vi "Generate_signal_names_based_on_sensor_names_v2_Core.vi"() -> ()   [LabVIEW 2011]
uses:
  <vilib>/addons/database/Connection.llb/DB Tools Open Connec (String).vi
  <vilib>/addons/database/NI_Database_API.lvlib
panel:
  in  "idtSignal OUT":u16[](array[numeric])=[0, 1, 2, 3, 4, 5, 6, 7, 8, 9, 10, 11, 12, 13, 14, 15, 16, 17, 18, 19, 20, 21, 22, 23, 24, 25, 26, 27, 28, 29, 30, 31, 32, 33, 34, 35, 36, 37, 38, 39, 40, 41, 42, 43, 44, 45, 46, 47, 48, 49, 50, 51, 52, 53, 54, 55, 56, 57, 58, 59, 60, 61, 62, 63, 64, 65, 66, 67, 68, 69, 70, 71, 72, 73, 74, 75, 76, 77, 78, 79, 80, 81, 82, 83, 84, 85, 86, 87, 88, 89, 90, 91, 92, 93, 94, 95, 96, 97, 98, 99, 100, 101, 102, 103, 104, 105, 106, 107, 108, 109, 110, 111, 112, 113, 114, 115, 116, 117, 118, 119, 120, 121, 122, 123, 124, 125, 126, 127, 128, 129, 130, 131, 132, 133, 134, 135, 136, 137, 138, 139, 140, 141, 142, 143, 144, 145, 146, 147, 148, 149, 150, 151, 152, 153, 154, 155, 156, 157, 158, 159, 160, 161, 162, 163, 164, 165, 166, 167, 168, 169, 170, 171, 172, 173, 174, 175, 176, 177, 178, 179, 180, 181, 182, 183, 184, 185, 186, 187, 188, 189, 190, 191, 192, 193, 194, 195, 196, 197, 198, 199, 200, 201, 202, 203, 204, 205, 206, 207, 208, 209, 210, 211, 212, 213, 214, 215, 216, 217, 218, 219, 220, 221, 222, 223, 224, 225, 226, 227, 228, 229, 230, 231, 232, 233, 234, 235, 236, 237, 238, 239, 240, 241, 242, 243, 244, 245, 246, 247, 248, 249, 250, 251, 252, 253, 254, 255, 256, 257, 258, 259, 260, 261, 262, 263, 264, 265, 266, 267, 268, 269, 270, 271, 272, 273, 274, 275, 276, 277, 278, 279, 280, 281, 282, 283, 284, 285, 286, 287, 288, 289, 290, 291, 292, 293, 294, 295, 296, 297, 298, 299, 300, 301, 302, 303, 304, 305, 306, 307, 308, 309, 310, 311, 312, 313, 314, 315, 316, 317, 318, 319, 320, 321, 322, 323, 324, 325, 326, 327, 328, 329, 330, 331, 332, 333, 334, 335, 336, 337, 338, 339, 340, 341, 342, 343, 344, 345, 346, 347, 348, 349, 350, 351, 352, 353, 354, 355, 356, 357, 358, 359, 360, 361, 362, 363, 364, 365, 366, 367, 368, 369, 370, 371, 372, 373, 374, 375, 376, 377, 378, 379, 380, 381, 382, 383, 384, 385, 386, 387, 388, 389, 390, 391, 392, 393, 394, 395, 396, 397, 398, 399, 400, 401, 402, 403, 404, 405, 406, 407, 408, 409, 410, 411, 412, 413, 414, 415, 416, 417, 418, 419, 420, 421, 422, 423, 424, 425, 426, 427, 428, 429, 430, 431, 432, 433, 434, 435, 437]
  out "error out":errorcluster={"status"=TRUE, "code"=-2147217900, "source"="NI_Database_API.lvlib:Cmd Execute.vi->NI_Database_API.lvlib:DB Tools Insert Data.vi->Generate_signal_names_based_on_sensor_names_v2_Erraring.vi<ERR>ADO Error: 0x80040E14\r\nException occured in Microsoft OLE DB Provider for ODBC Drivers: [MySQL][ODBC 5.1 Driver][mysqld-5.5.15]Duplicate entry '428' for key 'PRIMARY' in NI_Database_API.lvlib:Rec Create - Command.vi->NI_Database_API.lvlib:Cmd Execute.vi->NI_Database_API.lvlib:DB Tools Insert Data.vi->Generate_signal_names_based_on_sensor_names_v2_Erraring.vi"}
  in  "SignalNames":string[](array[string])=["Hitrost vrtenja 0 .RotSpeed.[1 impulz po obratu]", "Hitrost vrtenja 0 .DC.[V]", "Hitrost vrtenja 1 .RotSpeed.[100Hz]", "Hitrost vrtenja 1 .DC.[V]", "Relativne vibracije ZKL1 .s1.00A.[um]", "Relativne vibracije ZKL1 .s1.00Ph.[°]", "Relativne vibracije ZKL1 .s2.00A.[um]", "Relativne vibracije ZKL1 .s2.00Ph.[°]", "Relativne vibracije ZKL1 .s3.00A.[um]", "Relativne vibracije ZKL1 .s3.00Ph.[°]", "Relativne vibracije ZKL1 .Rest.[um]", "Relativne vibracije ZKL1 .DC.[um]", "Relativne vibracije ZKL1 .EqPeak.[um]", "Relativne vibracije ZKL1 &Relativne vibracije ZKL2 .Smax.[um]", "Relativne vibracije ZKL2 .s1.00A.[um]", "Relativne vibracije ZKL2 .s1.00Ph.[°]", "Relativne vibracije ZKL2 .s2.00A.[um]", "Relativne vibracije ZKL2 .s2.00Ph.[°]", "Relativne vibracije ZKL2 .s3.00A.[um]", "Relativne vibracije ZKL2 .s3.00Ph.[°]", "Relativne vibracije ZKL2 .Rest.[um]", "Relativne vibracije ZKL2 .DC.[um]", "Relativne vibracije ZKL2 .EqPeak.[um]", "Relativne vibracije SVL1 .s1.00A.[um]", "Relativne vibracije SVL1 .s1.00Ph.[°]", "Relativne vibracije SVL1 .s2.00A.[um]", "Relativne vibracije SVL1 .s2.00Ph.[°]", "Relativne vibracije SVL1 .s3.00A.[um]", "Relativne vibracije SVL1 .s3.00Ph.[°]", "Relativne vibracije SVL1 .Rest.[um]", "Relativne vibracije SVL1 .DC.[um]", "Relativne vibracije SVL1 .EqPeak.[um]", "Relativne vibracije SVL1 &Relativne vibracije SVL2 .Smax.[um]", "Relativne vibracije SVL2 .s1.00A.[um]", "Relativne vibracije SVL2 .s1.00Ph.[°]", "Relativne vibracije SVL2 .s2.00A.[um]", "Relativne vibracije SVL2 .s2.00Ph.[°]", "Relativne vibracije SVL2 .s3.00A.[um]", "Relativne vibracije SVL2 .s3.00Ph.[°]", "Relativne vibracije SVL2 .Rest.[um]", "Relativne vibracije SVL2 .DC.[um]", "Relativne vibracije SVL2 .EqPeak.[um]", "Relativne vibracije VVL1 .s1.00A.[um]", "Relativne vibracije VVL1 .s1.00Ph.[°]", "Relativne vibracije VVL1 .s2.00A.[um]", "Relativne vibracije VVL1 .s2.00Ph.[°]", "Relativne vibracije VVL1 .s3.00A.[um]", "Relativne vibracije VVL1 .s3.00Ph.[°]", "Relativne vibracije VVL1 .Rest.[um]", "Relativne vibracije VVL1 .DC.[um]", "Relativne vibracije VVL1 .EqPeak.[um]", "Relativne vibracije VVL1 &Relativne vibracije VVL2 .Smax.[um]", "Relativne vibracije VVL2 .s1.00A.[um]", "Relativne vibracije VVL2 .s1.00Ph.[°]", "Relativne vibracije VVL2 .s2.00A.[um]", "Relativne vibracije VVL2 .s2.00Ph.[°]", "Relativne vibracije VVL2 .s3.00A.[um]", "Relativne vibracije VVL2 .s3.00Ph.[°]", "Relativne vibracije VVL2 .Rest.[um]", "Relativne vibracije VVL2 .DC.[um]", "Relativne vibracije VVL2 .EqPeak.[um]", "Relativne vibracije TVL1 .s1.00A.[um]", "Relativne vibracije TVL1 .s1.00Ph.[°]", "Relativne vibracije TVL1 .s2.00A.[um]", "Relativne vibracije TVL1 .s2.00Ph.[°]", "Relativne vibracije TVL1 .s3.00A.[um]", "Relativne vibracije TVL1 .s3.00Ph.[°]", "Relativne vibracije TVL1 .Rest.[um]", "Relativne vibracije TVL1 .DC.[um]", "Relativne vibracije TVL1 .EqPeak.[um]", "Relativne vibracije TVL1 &Relativne vibracije TVL2 .Smax.[um]", "Relativne vibracije TVL2 .s1.00A.[um]", "Relativne vibracije TVL2 .s1.00Ph.[°]", "Relativne vibracije TVL2 .s2.00A.[um]", "Relativne vibracije TVL2 .s2.00Ph.[°]", "Relativne vibracije TVL2 .s3.00A.[um]", "Relativne vibracije TVL2 .s3.00Ph.[°]", "Relativne vibracije TVL2 .Rest.[um]", "Relativne vibracije TVL2 .DC.[um]", "Relativne vibracije TVL2 .EqPeak.[um]", "Absolutne vibracije ZKL1 .s1.00A.[mm/s]", "Absolutne vibracije ZKL1 .s1.00Ph.[°]", "Absolutne vibracije ZKL1 .s2.00A.[mm/s]", "Absolutne vibracije ZKL1 .s2.00Ph.[°]", "Absolutne vibracije ZKL1 .s3.00A.[mm/s]", "Absolutne vibracije ZKL1 .s3.00Ph.[°]", "Absolutne vibracije ZKL1 .Rest.[mm/s]", "Absolutne vibracije ZKL1 .RMS.[mm/s]", "Absolutne vibracije ZKL1 .DC.[mm/s]", "Absolutne vibracije ZKL2 .s1.00A.[mm/s]", "Absolutne vibracije ZKL2 .s1.00Ph.[°]", "Absolutne vibracije ZKL2 .s2.00A.[mm/s]", "Absolutne vibracije ZKL2 .s2.00Ph.[°]", "Absolutne vibracije ZKL2 .s3.00A.[mm/s]", "Absolutne vibracije ZKL2 .s3.00Ph.[°]", "Absolutne vibracije ZKL2 .Rest.[mm/s]", "Absolutne vibracije ZKL2 .RMS.[mm/s]", "Absolutne vibracije ZKL2 .DC.[mm/s]", "Absolutne vibracije SVL1 .s1.00A.[mm/s]", "Absolutne vibracije SVL1 .s1.00Ph.[°]", "Absolutne vibracije SVL1 .s2.00A.[mm/s]", "Absolutne vibracije SVL1 .s2.00Ph.[°]", "Absolutne vibracije SVL1 .s3.00A.[mm/s]", "Absolutne vibracije SVL1 .s3.00Ph.[°]", "Absolutne vibracije SVL1 .Rest.[mm/s]", "Absolutne vibracije SVL1 .RMS.[mm/s]", "Absolutne vibracije SVL1 .DC.[mm/s]", "Absolutne vibracije SVL2 .s1.00A.[mm/s]", "Absolutne vibracije SVL2 .s1.00Ph.[°]", "Absolutne vibracije SVL2 .s2.00A.[mm/s]", "Absolutne vibracije SVL2 .s2.00Ph.[°]", "Absolutne vibracije SVL2 .s3.00A.[mm/s]", "Absolutne vibracije SVL2 .s3.00Ph.[°]", "Absolutne vibracije SVL2 .Rest.[mm/s]", "Absolutne vibracije SVL2 .RMS.[mm/s]", "Absolutne vibracije SVL2 .DC.[mm/s]", "Absolutne vibracije VVL1 .s1.00A.[mm/s]", "Absolutne vibracije VVL1 .s1.00Ph.[°]", "Absolutne vibracije VVL1 .s2.00A.[mm/s]", "Absolutne vibracije VVL1 .s2.00Ph.[°]", "Absolutne vibracije VVL1 .s3.00A.[mm/s]", "Absolutne vibracije VVL1 .s3.00Ph.[°]", "Absolutne vibracije VVL1 .Rest.[mm/s]", "Absolutne vibracije VVL1 .RMS.[mm/s]", "Absolutne vibracije VVL1 .DC.[mm/s]", "Absolutne vibracije VVL1 .s1.00A.[mm/s]", "Absolutne vibracije VVL1 .s1.00Ph.[°]", "Absolutne vibracije VVL1 .s2.00A.[mm/s]", "Absolutne vibracije VVL1 .s2.00Ph.[°]", "Absolutne vibracije VVL1 .s3.00A.[mm/s]", "Absolutne vibracije VVL1 .s3.00Ph.[°]", "Absolutne vibracije VVL1 .Rest.[mm/s]", "Absolutne vibracije VVL1 .RMS.[mm/s]", "Absolutne vibracije VVL1 .DC.[mm/s]", "Absolutne vibracije TVL1 .s1.00A.[mm/s]", "Absolutne vibracije TVL1 .s1.00Ph.[°]", "Absolutne vibracije TVL1 .s2.00A.[mm/s]", "Absolutne vibracije TVL1 .s2.00Ph.[°]", "Absolutne vibracije TVL1 .s3.00A.[mm/s]", "Absolutne vibracije TVL1 .s3.00Ph.[°]", "Absolutne vibracije TVL1 .Rest.[mm/s]", "Absolutne vibracije TVL1 .RMS.[mm/s]", "Absolutne vibracije TVL1 .DC.[mm/s]", "Absolutne vibracije TVL2 .s1.00A.[mm/s]", "Absolutne vibracije TVL2 .s1.00Ph.[°]", "Absolutne vibracije TVL2 .s2.00A.[mm/s]", "Absolutne vibracije TVL2 .s2.00Ph.[°]", "Absolutne vibracije TVL2 .s3.00A.[mm/s]", "Absolutne vibracije TVL2 .s3.00Ph.[°]", "Absolutne vibracije TVL2 .Rest.[mm/s]", "Absolutne vibracije TVL2 .RMS.[mm/s]", "Absolutne vibracije TVL2 .DC.[mm/s]", "Aksialni pomik  AxP1 .DC.[um]", "Aksialni pomik  AxP2 .DC.[um]", "Absolutne vibracije paketa VP1 .RMS.[mm/s]", "Absolutne vibracije paketa VP1 .s20.00A.[mm/s]", "Absolutne vibracije paketa VP1 .s40.00A.[mm/s]", "Absolutne vibracije paketa VP1 .s60.00A.[mm/s]", "Absolutne vibracije paketa VP1 .Rest.[mm/s]", "Absolutne vibracije paketa VP2 .RMS.[mm/s]", "Absolutne vibracije paketa VP2 .s20.00A.[mm/s]", "Absolutne vibracije paketa VP2 .s40.00A.[mm/s]", "Absolutne vibracije paketa VP2 .s60.00A.[mm/s]", "Absolutne vibracije paketa VP2 .Rest.[mm/s]", "Zracna reža zgoraj, dajalec 1 .MinPole01.[mm]", "Zracna reža zgoraj, dajalec 1 .MinPole02.[mm]", "Zracna reža zgoraj, dajalec 1 .MinPole03.[mm]", "Zracna reža zgoraj, dajalec 1 .MinPole04.[mm]", "Zracna reža zgoraj, dajalec 1 .MinPole05.[mm]", "Zracna reža zgoraj, dajalec 1 .MinPole06.[mm]", "Zracna reža zgoraj, dajalec 1 .MinPole07.[mm]", "Zracna reža zgoraj, dajalec 1 .MinPole08.[mm]", "Zracna reža zgoraj, dajalec 1 .MinPole09.[mm]", "Zracna reža zgoraj, dajalec 1 .MinPole10.[mm]", "Zracna reža zgoraj, dajalec 1 .MinPole11.[mm]", "Zracna reža zgoraj, dajalec 1 .MinPole12.[mm]", "Zracna reža zgoraj, dajalec 1 .MinPole13.[mm]", "Zracna reža zgoraj, dajalec 1 .MinPole14.[mm]", "Zracna reža zgoraj, dajalec 1 .MinPole15.[mm]", "Zracna reža zgoraj, dajalec 1 .MinPole16.[mm]", "Zracna reža zgoraj, dajalec 1 .MinPole17.[mm]", "Zracna reža zgoraj, dajalec 1 .MinPole18.[mm]", "Zracna reža zgoraj, dajalec 1 .MinPole19.[mm]", "Zracna reža zgoraj, dajalec 1 .MinPole20.[mm]", "Zracna reža zgoraj, dajalec 1 .MinExtremaMin.[mm]", "Zracna reža zgoraj, dajalec 1 .MinExtremaMinPoleNum.[Number]", "Zracna reža zgoraj, dajalec 1 .MaxExtremaMin.[mm]", "Zracna reža zgoraj, dajalec 1 .MaxExtremaMinPoleNum.[Number]", "Zracna reža zgoraj, dajalec 1 .DCExtremaMin.[mm]", "Zracna reža zgoraj, dajalec 1 .MaxDiff.[mm]", "Zracna reža zgoraj, dajalec 1 .MaxDiffPoleNum.[Number]", "Zracna reža zgoraj, dajalec 1 .Max Diff Pole Number.[mm]", "Zracna reža zgoraj, dajalec 1 .s1.00A.[mm]", "Zracna reža zgoraj, dajalec 1 .s1.00Ph.[°]", "Zracna reža zgoraj, dajalec 1 .s2.00A.[mm]", "Zracna reža zgoraj, dajalec 1 .s2.00Ph.[°]", "Zracna reža zgoraj, dajalec 1 .DC.[mm]", "Zracna reža zgoraj, dajalec 2 .MinPole01.[mm]", "Zracna reža zgoraj, dajalec 2 .MinPole02.[mm]", "Zracna reža zgoraj, dajalec 2 .MinPole03.[mm]", "Zracna reža zgoraj, dajalec 2 .MinPole04.[mm]", "Zracna reža zgoraj, dajalec 2 .MinPole05.[mm]", "Zracna reža zgoraj, dajalec 2 .MinPole06.[mm]", "Zracna reža zgoraj, dajalec 2 .MinPole07.[mm]", "Zracna reža zgoraj, dajalec 2 .MinPole08.[mm]", "Zracna reža zgoraj, dajalec 2 .MinPole09.[mm]", "Zracna reža zgoraj, dajalec 2 .MinPole10.[mm]", "Zracna reža zgoraj, dajalec 2 .MinPole11.[mm]", "Zracna reža zgoraj, dajalec 2 .MinPole12.[mm]", "Zracna reža zgoraj, dajalec 2 .MinPole13.[mm]", "Zracna reža zgoraj, dajalec 2 .MinPole14.[mm]", "Zracna reža zgoraj, dajalec 2 .MinPole15.[mm]", "Zracna reža zgoraj, dajalec 2 .MinPole16.[mm]", "Zracna reža zgoraj, dajalec 2 .MinPole17.[mm]", "Zracna reža zgoraj, dajalec 2 .MinPole18.[mm]", "Zracna reža zgoraj, dajalec 2 .MinPole19.[mm]", "Zracna reža zgoraj, dajalec 2 .MinPole20.[mm]", "Zracna reža zgoraj, dajalec 2 .MinExtremaMin.[mm]", "Zracna reža zgoraj, dajalec 2 .MinExtremaMinPoleNum.[Number]", "Zracna reža zgoraj, dajalec 2 .MaxExtremaMin.[mm]", "Zracna reža zgoraj, dajalec 2 .MaxExtremaMinPoleNum.[Number]", "Zracna reža zgoraj, dajalec 2 .DCExtremaMin.[mm]", "Zracna reža zgoraj, dajalec 2 .MaxDiff.[mm]", "Zracna reža zgoraj, dajalec 2 .MaxDiffPoleNum.[Number]", "Zracna reža zgoraj, dajalec 2 .Max Diff Pole Number.[mm]", "Zracna reža zgoraj, dajalec 2 .s1.00A.[mm]", "Zracna reža zgoraj, dajalec 2 .s1.00Ph.[°]", "Zracna reža zgoraj, dajalec 2 .s2.00A.[mm]", "Zracna reža zgoraj, dajalec 2 .s2.00Ph.[°]", "Zracna reža zgoraj, dajalec 2 .DC.[mm]", "Magnetno polje, dajalec zgoraj .MaxPole01.[T]", "Magnetno polje, dajalec zgoraj .MaxPole02.[T]", "Magnetno polje, dajalec zgoraj .MaxPole03.[T]", "Magnetno polje, dajalec zgoraj .MaxPole04.[T]", "Magnetno polje, dajalec zgoraj .MaxPole05.[T]", "Magnetno polje, dajalec zgoraj .MaxPole06.[T]", "Magnetno polje, dajalec zgoraj .MaxPole07.[T]", "Magnetno polje, dajalec zgoraj .MaxPole08.[T]", "Magnetno polje, dajalec zgoraj .MaxPole09.[T]", "Magnetno polje, dajalec zgoraj .MaxPole10.[T]", "Magnetno polje, dajalec zgoraj .MaxPole11.[T]", "Magnetno polje, dajalec zgoraj .MaxPole12.[T]", "Magnetno polje, dajalec zgoraj .MaxPole13.[T]", "Magnetno polje, dajalec zgoraj .MaxPole14.[T]", "Magnetno polje, dajalec zgoraj .MaxPole15.[T]", "Magnetno polje, dajalec zgoraj .MaxPole16.[T]", "Magnetno polje, dajalec zgoraj .MaxPole17.[T]", "Magnetno polje, dajalec zgoraj .MaxPole18.[T]", "Magnetno polje, dajalec zgoraj .MaxPole19.[T]", "Magnetno polje, dajalec zgoraj .MaxPole20.[T]", "Magnetno polje, dajalec zgoraj .MinExtremaMax.[T]", "Magnetno polje, dajalec zgoraj .MinExtremaMaxPoleNum.[Number]", "Magnetno polje, dajalec zgoraj .MaxExtremaMax.[T]", "Magnetno polje, dajalec zgoraj .MaxExtremaMaxPoleNum.[Number]", "Magnetno polje, dajalec zgoraj .DCExtremaMax.[T]", "Magnetno polje, dajalec zgoraj .MaxDiff.[T]", "Magnetno polje, dajalec zgoraj .MaxDiffPoleNum.[Number]", "Magnetno polje, dajalec zgoraj .Max Diff Pole Number.[T]", "Hitrost vrtenja 1 &Napetost generatorja faza R .LoadAngleDelta.[100Hz]", "Napetost generatorja faza R - G1 .ActivePowerIntegration.[kV]", "Napetost generatorja faza R - G1 .ReactivePowerIntegration.[kV]", "Napetost generatorja faza R - G1 .ApparentPower.[kV]", "Napetost generatorja faza R - G1 .Ampl@Freq.[kV]", "Napetost generatorja faza S - G1 .Ampl@Freq.[kV]", "Napetost generatorja faza T - G1 .Ampl@Freq.[kV]", "Tok generatorja faza R - G1 .Ampl@Freq.[kA]", "Tok generatorja faza S - G1 .Ampl@Freq.[kA]", "Tok generatorja faza T - G1 .Ampl@Freq.[kA]", "Napetost za blok transformatorjem faza R - G1 .Ampl@Freq.[kV]", "Napetost za blok transformatorjem faza S - G1 .Ampl@Freq.[kV]", "Napetost za blok transformatorjem faza T - G1 .Ampl@Freq.[kV]", "Tok za blok transformatorjem faza R - G1 .Ampl@Freq.[A]", "Tok za blok transformatorjem faza S - G1 .Ampl@Freq.[A]", "Tok za blok transformatorjem faza T - G1 .Ampl@Freq.[A]", "Napetost generatorja faza R - G1 .SignalFrequency.[Hz]", "Napetost generatorja faza S - G1 .SignalFrequency.[Hz]", "Napetost generatorja faza T - G1 .SignalFrequency.[Hz]", "Tok generatorja faza R - G1 .SignalFrequency.[Hz]", "Tok generatorja faza S - G1 .SignalFrequency.[Hz]", "Tok generatorja faza T - G1 .SignalFrequency.[Hz]", "Napetost za blok transformatorjem faza R - G1 .SignalFrequency.[Hz]", "Napetost za blok transformatorjem faza S - G1 .SignalFrequency.[Hz]", "Napetost za blok transformatorjem faza T - G1 .SignalFrequency.[Hz]", "Tok za blok transformatorjem faza R - G1 .SignalFrequency.[Hz]", "Tok za blok transformatorjem faza S - G1 .SignalFrequency.[Hz]", "Tok za blok transformatorjem faza T - G1 .SignalFrequency.[Hz]", "Napetost generatorja faza R - G1 .THD.[%]", "Napetost generatorja faza S - G1 .THD.[%]", "Napetost generatorja faza T - G1 .THD.[%]", "Tok generatorja faza R - G1 .THD.[%]", "Tok generatorja faza S - G1 .THD.[%]", "Tok generatorja faza T - G1 .THD.[%]", "Napetost za blok transformatorjem faza R - G1 .THD.[%]", "Napetost za blok transformatorjem faza S - G1 .THD.[%]", "Napetost za blok transformatorjem faza T - G1 .THD.[%]", "Tok za blok transformatorjem faza R - G1 .THD.[%]", "Tok za blok transformatorjem faza S - G1 .THD.[%]", "Tok za blok transformatorjem faza T - G1 .THD.[%]", "Napetost generatorja faza R - G1 &Napetost generatorja faza S - G1 .PhaseDifference.[°]", "Napetost generatorja faza S - G1 &Napetost generatorja faza T - G1 .PhaseDifference.[°]", "Napetost generatorja faza T - G1 &Napetost generatorja faza R - G1 .PhaseDifference.[°]", "Tok generatorja faza R - G1 &Tok generatorja faza S - G1 .PhaseDifference.[°]", "Tok generatorja faza S - G1 &Tok generatorja faza T - G1 .PhaseDifference.[°]", "Tok generatorja faza T - G1 &Tok generatorja faza R - G1 .PhaseDifference.[°]", "Napetost za blok transformatorjem faza R - G1 &Napetost za blok transformatorjem faza S - G1 .PhaseDifference.[°]", "Napetost za blok transformatorjem faza S - G1 &Napetost za blok transformatorjem faza T - G1 .PhaseDifference.[°]", "Napetost za blok transformatorjem faza T - G1 &Napetost za blok transformatorjem faza R - G1 .PhaseDifference.[°]", "Tok za blok transformatorjem faza R - G1 &Tok za blok transformatorjem faza S - G1 .PhaseDifference.[°]", "Tok za blok transformatorjem faza S - G1 &Tok za blok transformatorjem faza T - G1 .PhaseDifference.[°]", "Tok za blok transformatorjem faza T - G1 &Tok za blok transformatorjem faza R - G1 .PhaseDifference.[°]", "Napetost generatorja faza R - G1 .CosFi.[%]", "Napetost generatorja faza R - G1 .TotalTHD.[%]", "Tok generatorja faza R - G1 .TotalTHD.[%]", "Napetost za blok transformatorjem faza R - G1 .TotalTHD.[%]", "Tok za blok transformatorjem faza R - G1 .TotalTHD.[%]", "ModbusData_000", "ModbusData_001", "ModbusData_002", "ModbusData_003", "ModbusData_004", "ModbusData_005", "ModbusData_006", "ModbusData_007", "ModbusData_008", "ModbusData_009", "ModbusData_010", "ModbusData_011", "ModbusData_012", "ModbusData_013", "ModbusData_014", "ModbusData_015", "ModbusData_016", "ModbusData_017", "ModbusData_018", "ModbusData_019", "ModbusData_020", "ModbusData_021", "ModbusData_022", "ModbusData_023", "ModbusData_024", "ModbusData_025", "ModbusData_026", "ModbusData_027", "ModbusData_028", "ModbusData_029", "ModbusData_030", "ModbusData_031", "ModbusData_032", "ModbusData_033", "ModbusData_034", "ModbusData_035", "ModbusData_036", "ModbusData_037", "ModbusData_038", "ModbusData_039", "ModbusData_040", "ModbusData_041", "ModbusData_042", "ModbusData_043", "ModbusData_044", "ModbusData_045", "ModbusData_046", "ModbusData_047", "ModbusData_048", "ModbusData_049", "ModbusData_050", "ModbusData_051", "ModbusData_052", "ModbusData_053", "ModbusData_054", "ModbusData_055", "ModbusData_056", "ModbusData_057", "ModbusData_058", "ModbusData_059", "ModbusData_060", "ModbusData_061", "ModbusData_062", "ModbusData_063", "ModbusData_064", "ModbusData_065", "ModbusData_066", "ModbusData_067", "ModbusData_068", "ModbusData_069", "ModbusData_070", "ModbusData_071", "ModbusData_072", "ModbusData_073", "ModbusData_074", "ModbusData_075", "ModbusData_076", "ModbusData_077", "ModbusData_078", "ModbusData_079", "ModbusData_080", "ModbusData_081", "ModbusData_082", "ModbusData_083", "ModbusData_084", "ModbusData_085", "ModbusData_086", "ModbusData_087", "ModbusData_088", "ModbusData_089", "ModbusData_090", "ModbusData_091", "ModbusData_092", "ModbusData_093", "ModbusData_094", "ModbusData_095", "ModbusData_096", "ModbusData_097", "ModbusData_098", "ModbusData_099", "Absolutne vibracije paketa VP1 .DC.[mm/s]", "Absolutne vibracije paketa VP2 .DC.[mm/s]", "Absolutne vibracije paketa VP1 .EqPeak.[mm/s]", "Absolutne vibracije paketa VP2 .EqPeak.[mm/s]", "Magnetno polje, dajalec zgoraj .DC.[T]", "Absolutne vibracije ZKL1 .EqPeak.[mm/s]", "Absolutne vibracije ZKL2 .EqPeak.[mm/s]", "Absolutne vibracije SVL1 .EqPeak.[mm/s]", "Absolutne vibracije SVL2 .EqPeak.[mm/s]", "Absolutne vibracije VVL1 .EqPeak.[mm/s]", "Absolutne vibracije VVL1 .EqPeak.[mm/s]", "Absolutne vibracije TVL1 .EqPeak.[mm/s]", "Absolutne vibracije TVL2 .EqPeak.[mm/s]", "Magnetno polje, dajalec zgoraj .EqPeak.[T]", "Relativne vibracije ZKL1 &Relativne vibracije ZKL2 .SP2Pmax.[um]", "Relativne vibracije SVL1 &Relativne vibracije SVL2 .SP2Pmax.[um]", "Relativne vibracije VVL1 &Relativne vibracije VVL2 .SP2Pmax.[um]", "Relativne vibracije TVL1 &Relativne vibracije TVL2 .SP2Pmax.[um]", "Magnetno polje, dajalec zgoraj .RMS.[T]", "Magnetno polje, dajalec zgoraj .EqPeak.[T]", "Napetost generatorja faza R .s10.00A.[kV]", "Napetost generatorja faza R .s10.00Ph.[°]"]
  in  "SignalLabels":string[](array[string])=["TRG000.RotSpeed", "TRG000.DC", "TRG001.RotSpeed", "TRG001.DC", "RV000.s1.00A", "RV000.s1.00Ph", "RV000.s2.00A", "RV000.s2.00Ph", "RV000.s3.00A", "RV000.s3.00Ph", "RV000.Rest", "RV000.DC", "RV000.EqPeak", "RV000&RV001.Smax", "RV001.s1.00A", "RV001.s1.00Ph", "RV001.s2.00A", "RV001.s2.00Ph", "RV001.s3.00A", "RV001.s3.00Ph", "RV001.Rest", "RV001.DC", "RV001.EqPeak", "RV002.s1.00A", "RV002.s1.00Ph", "RV002.s2.00A", "RV002.s2.00Ph", "RV002.s3.00A", "RV002.s3.00Ph", "RV002.Rest", "RV002.DC", "RV002.EqPeak", "RV002&RV003.Smax", "RV003.s1.00A", "RV003.s1.00Ph", "RV003.s2.00A", "RV003.s2.00Ph", "RV003.s3.00A", "RV003.s3.00Ph", "RV003.Rest", "RV003.DC", "RV003.EqPeak", "RV004.s1.00A", "RV004.s1.00Ph", "RV004.s2.00A", "RV004.s2.00Ph", "RV004.s3.00A", "RV004.s3.00Ph", "RV004.Rest", "RV004.DC", "RV004.EqPeak", "RV004&RV005.Smax", "RV005.s1.00A", "RV005.s1.00Ph", "RV005.s2.00A", "RV005.s2.00Ph", "RV005.s3.00A", "RV005.s3.00Ph", "RV005.Rest", "RV005.DC", "RV005.EqPeak", "RV006.s1.00A", "RV006.s1.00Ph", "RV006.s2.00A", "RV006.s2.00Ph", "RV006.s3.00A", "RV006.s3.00Ph", "RV006.Rest", "RV006.DC", "RV006.EqPeak", "RV006&RV007.Smax", "RV007.s1.00A", "RV007.s1.00Ph", "RV007.s2.00A", "RV007.s2.00Ph", "RV007.s3.00A", "RV007.s3.00Ph", "RV007.Rest", "RV007.DC", "RV007.EqPeak", "AV000.s1.00A", "AV000.s1.00Ph", "AV000.s2.00A", "AV000.s2.00Ph", "AV000.s3.00A", "AV000.s3.00Ph", "AV000.Rest", "AV000.RMS", "AV000.DC", "AV001.s1.00A", "AV001.s1.00Ph", "AV001.s2.00A", "AV001.s2.00Ph", "AV001.s3.00A", "AV001.s3.00Ph", "AV001.Rest", "AV001.RMS", "AV001.DC", "AV002.s1.00A", "AV002.s1.00Ph", "AV002.s2.00A", "AV002.s2.00Ph", "AV002.s3.00A", "AV002.s3.00Ph", "AV002.Rest", "AV002.RMS", "AV002.DC", "AV003.s1.00A", "AV003.s1.00Ph", "AV003.s2.00A", "AV003.s2.00Ph", "AV003.s3.00A", "AV003.s3.00Ph", "AV003.Rest", "AV003.RMS", "AV003.DC", "AV004.s1.00A", "AV004.s1.00Ph", "AV004.s2.00A", "AV004.s2.00Ph", "AV004.s3.00A", "AV004.s3.00Ph", "AV004.Rest", "AV004.RMS", "AV004.DC", "AV005.s1.00A", "AV005.s1.00Ph", "AV005.s2.00A", "AV005.s2.00Ph", "AV005.s3.00A", "AV005.s3.00Ph", "AV005.Rest", "AV005.RMS", "AV005.DC", "AV006.s1.00A", "AV006.s1.00Ph", "AV006.s2.00A", "AV006.s2.00Ph", "AV006.s3.00A", "AV006.s3.00Ph", "AV006.Rest", "AV006.RMS", "AV006.DC", "AV007.s1.00A", "AV007.s1.00Ph", "AV007.s2.00A", "AV007.s2.00Ph", "AV007.s3.00A", "AV007.s3.00Ph", "AV007.Rest", "AV007.RMS", "AV007.DC", "AXD000.DC", "AXD001.DC", "AV008.RMS", "AV008.s20.00A", "AV008.s40.00A", "AV008.s60.00A", "AV008.Rest", "AV009.RMS", "AV009.s20.00A", "AV009.s40.00A", "AV009.s60.00A", "AV009.Rest", "AG000.MinPole01", "AG000.MinPole02", "AG000.MinPole03", "AG000.MinPole04", "AG000.MinPole05", "AG000.MinPole06", "AG000.MinPole07", "AG000.MinPole08", "AG000.MinPole09", "AG000.MinPole10", "AG000.MinPole11", "AG000.MinPole12", "AG000.MinPole13", "AG000.MinPole14", "AG000.MinPole15", "AG000.MinPole16", "AG000.MinPole17", "AG000.MinPole18", "AG000.MinPole19", "AG000.MinPole20", "AG000.MinExtremaMin", "AG000.MinExtremaMinPoleNum", "AG000.MaxExtremaMin", "AG000.MaxExtremaMinPoleNum", "AG000.DCExtremaMin", "AG000.MaxDiff", "AG000.MaxDiffPoleNum", "AG000.Max Diff Pole Number", "AG000.s1.00A", "AG000.s1.00Ph", "AG000.s2.00A", "AG000.s2.00Ph", "AG000.DC", "AG001.MinPole01", "AG001.MinPole02", "AG001.MinPole03", "AG001.MinPole04", "AG001.MinPole05", "AG001.MinPole06", "AG001.MinPole07", "AG001.MinPole08", "AG001.MinPole09", "AG001.MinPole10", "AG001.MinPole11", "AG001.MinPole12", "AG001.MinPole13", "AG001.MinPole14", "AG001.MinPole15", "AG001.MinPole16", "AG001.MinPole17", "AG001.MinPole18", "AG001.MinPole19", "AG001.MinPole20", "AG001.MinExtremaMin", "AG001.MinExtremaMinPoleNum", "AG001.MaxExtremaMin", "AG001.MaxExtremaMinPoleNum", "AG001.DCExtremaMin", "AG001.MaxDiff", "AG001.MaxDiffPoleNum", "AG001.Max Diff Pole Number", "AG001.s1.00A", "AG001.s1.00Ph", "AG001.s2.00A", "AG001.s2.00Ph", "AG001.DC", "MX000.MaxPole01", "MX000.MaxPole02", "MX000.MaxPole03", "MX000.MaxPole04", "MX000.MaxPole05", "MX000.MaxPole06", "MX000.MaxPole07", "MX000.MaxPole08", "MX000.MaxPole09", "MX000.MaxPole10", "MX000.MaxPole11", "MX000.MaxPole12", "MX000.MaxPole13", "MX000.MaxPole14", "MX000.MaxPole15", "MX000.MaxPole16", "MX000.MaxPole17", "MX000.MaxPole18", "MX000.MaxPole19", "MX000.MaxPole20", "MX000.MinExtremaMax", "MX000.MinExtremaMaxPoleNum", "MX000.MaxExtremaMax", "MX000.MaxExtremaMaxPoleNum", "MX000.DCExtremaMax", "MX000.MaxDiff", "MX000.MaxDiffPoleNum", "MX000.Max Diff Pole Number", "TRG001&PROC000.LoadAngleDelta", "VOL000.ActivePowerIntegration", "VOL000.ReactivePowerIntegration", "VOL000.ApparentPower", "VOL000.Ampl@Freq", "VOL001.Ampl@Freq", "VOL002.Ampl@Freq", "CURR000.Ampl@Freq", "CURR001.Ampl@Freq", "CURR002.Ampl@Freq", "VOL004.Ampl@Freq", "VOL005.Ampl@Freq", "VOL006.Ampl@Freq", "CURR004.Ampl@Freq", "CURR005.Ampl@Freq", "CURR006.Ampl@Freq", "VOL000.SignalFrequency", "VOL001.SignalFrequency", "VOL002.SignalFrequency", "CURR000.SignalFrequency", "CURR001.SignalFrequency", "CURR002.SignalFrequency", "VOL004.SignalFrequency", "VOL005.SignalFrequency", "VOL006.SignalFrequency", "CURR004.SignalFrequency", "CURR005.SignalFrequency", "CURR006.SignalFrequency", "VOL000.THD", "VOL001.THD", "VOL002.THD", "CURR000.THD", "CURR001.THD", "CURR002.THD", "VOL004.THD", "VOL005.THD", "VOL006.THD", "CURR004.THD", "CURR005.THD", "CURR006.THD", "VOL000&VOL001.PhaseDifference", "VOL001&VOL002.PhaseDifference", "VOL002&VOL000.PhaseDifference", "CURR000&CURR001.PhaseDifference", "CURR001&CURR002.PhaseDifference", "CURR002&CURR000.PhaseDifference", "VOL004&VOL005.PhaseDifference", "VOL005&VOL006.PhaseDifference", "VOL006&VOL004.PhaseDifference", "CURR004&CURR005.PhaseDifference", "CURR005&CURR006.PhaseDifference", "CURR006&CURR004.PhaseDifference", "VOL000.CosFi", "VOL000.TotalTHD", "CURR000.TotalTHD", "VOL004.TotalTHD", "CURR004.TotalTHD", "ModbusData_000", "ModbusData_001", "ModbusData_002", "ModbusData_003", "ModbusData_004", "ModbusData_005", "ModbusData_006", "ModbusData_007", "ModbusData_008", "ModbusData_009", "ModbusData_010", "ModbusData_011", "ModbusData_012", "ModbusData_013", "ModbusData_014", "ModbusData_015", "ModbusData_016", "ModbusData_017", "ModbusData_018", "ModbusData_019", "ModbusData_020", "ModbusData_021", "ModbusData_022", "ModbusData_023", "ModbusData_024", "ModbusData_025", "ModbusData_026", "ModbusData_027", "ModbusData_028", "ModbusData_029", "ModbusData_030", "ModbusData_031", "ModbusData_032", "ModbusData_033", "ModbusData_034", "ModbusData_035", "ModbusData_036", "ModbusData_037", "ModbusData_038", "ModbusData_039", "ModbusData_040", "ModbusData_041", "ModbusData_042", "ModbusData_043", "ModbusData_044", "ModbusData_045", "ModbusData_046", "ModbusData_047", "ModbusData_048", "ModbusData_049", "ModbusData_050", "ModbusData_051", "ModbusData_052", "ModbusData_053", "ModbusData_054", "ModbusData_055", "ModbusData_056", "ModbusData_057", "ModbusData_058", "ModbusData_059", "ModbusData_060", "ModbusData_061", "ModbusData_062", "ModbusData_063", "ModbusData_064", "ModbusData_065", "ModbusData_066", "ModbusData_067", "ModbusData_068", "ModbusData_069", "ModbusData_070", "ModbusData_071", "ModbusData_072", "ModbusData_073", "ModbusData_074", "ModbusData_075", "ModbusData_076", "ModbusData_077", "ModbusData_078", "ModbusData_079", "ModbusData_080", "ModbusData_081", "ModbusData_082", "ModbusData_083", "ModbusData_084", "ModbusData_085", "ModbusData_086", "ModbusData_087", "ModbusData_088", "ModbusData_089", "ModbusData_090", "ModbusData_091", "ModbusData_092", "ModbusData_093", "ModbusData_094", "ModbusData_095", "ModbusData_096", "ModbusData_097", "ModbusData_098", "ModbusData_099", "AV008.DC", "AV009.DC", "AV008.EqPeak", "AV009.EqPeak", "MX000.DC", "AV000.EqPeak", "AV001.EqPeak", "AV002.EqPeak", "AV003.EqPeak", "AV004.EqPeak", "AV005.EqPeak", "AV006.EqPeak", "AV007.EqPeak", "MX000.EqPeak", "RV000&RV001.SP2Pmax", "RV002&RV003.SP2Pmax", "RV004&RV005.SP2Pmax", "RV006&RV007.SP2Pmax", "MX000.RMS", "MX000.EqPeak", "PROC000.s10.00A", "PROC000.s10.00Ph"]
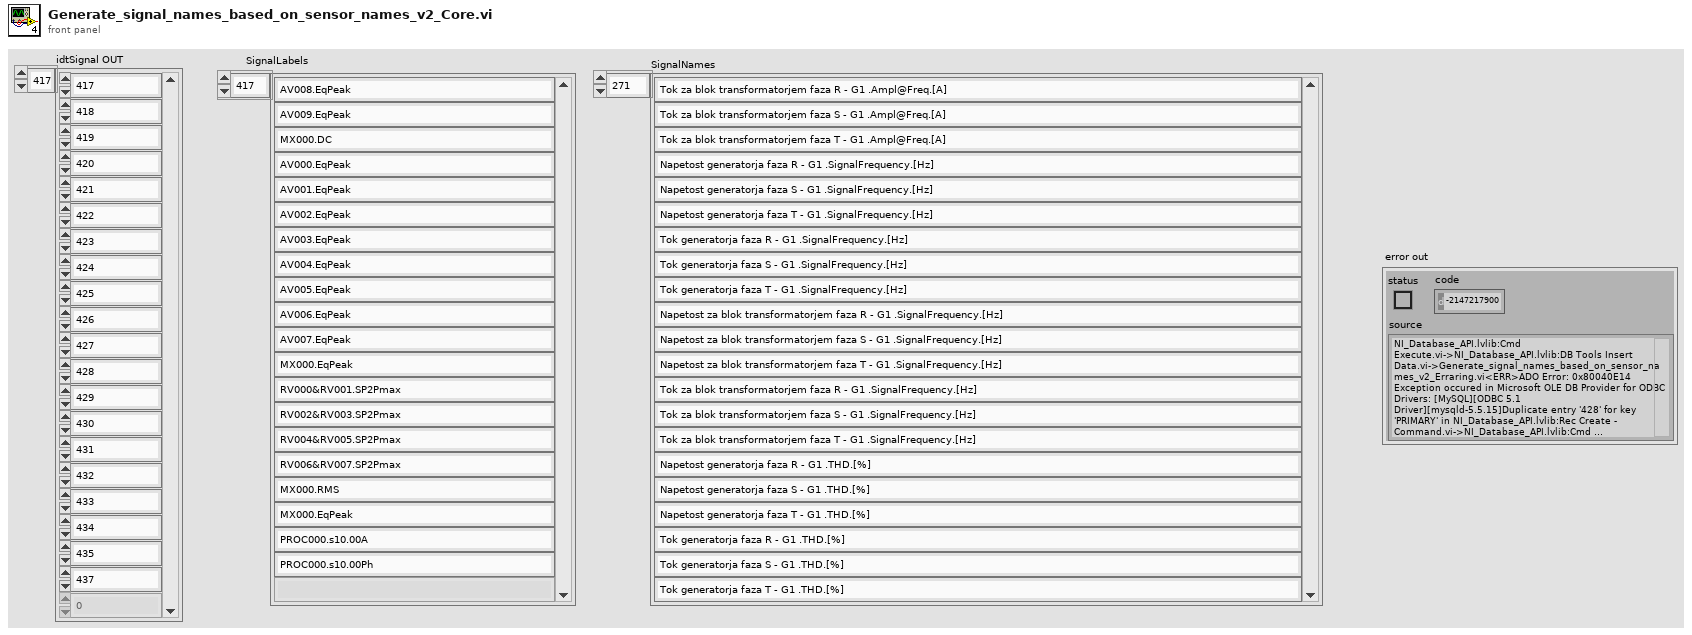
[diagram p1: front panel]
types:
  T1 = typedef "NI_Database_API.lvlib/Conn ObjectReference.ctl" = refnum<k1>
  T2 = cluster{"data":u16, "data":string, "result string":string, "String":string}
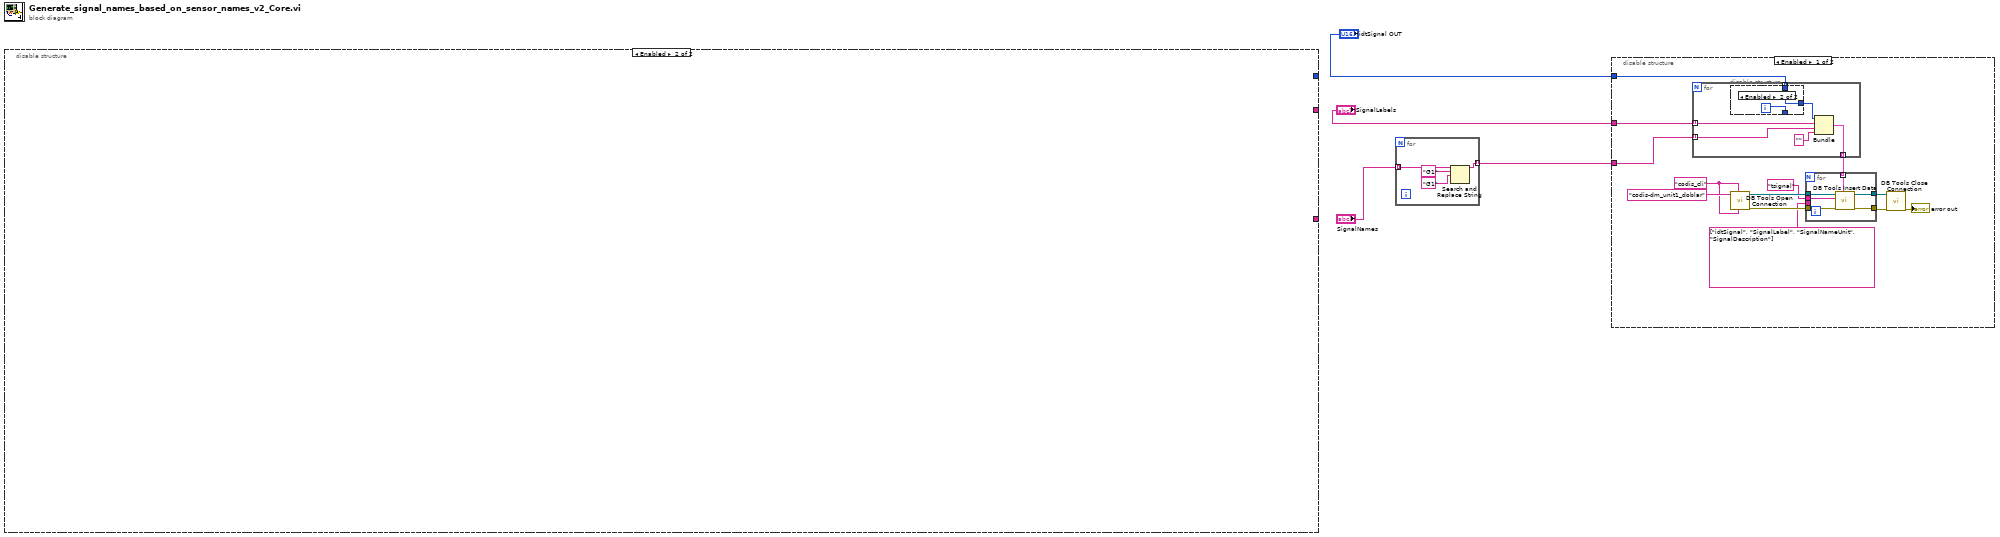
[diagram p0: block diagram]
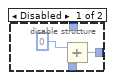
[diagram p2: hidden frame]
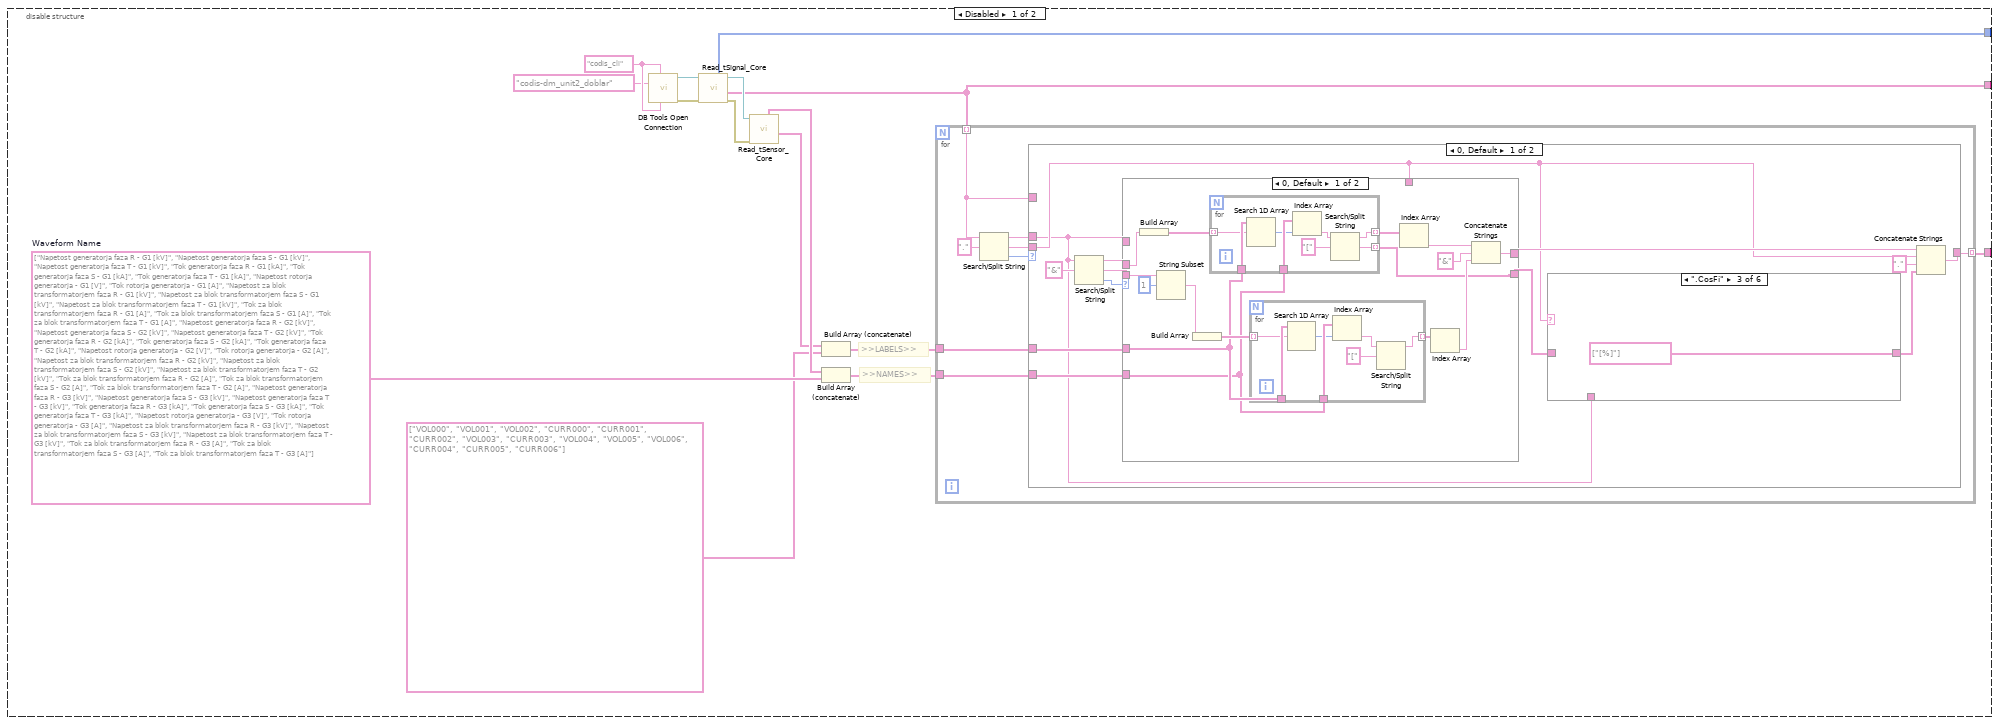
[diagram p4: hidden frame]
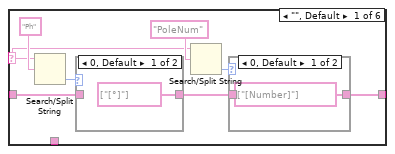
[diagram p5: hidden frame]
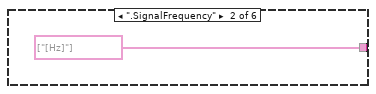
[diagram p8: hidden frame]
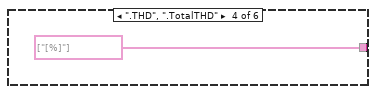
[diagram p9: hidden frame]
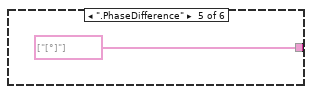
[diagram p10: hidden frame]
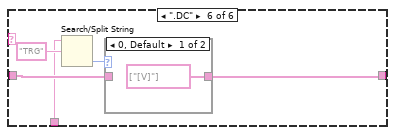
[diagram p11: hidden frame]
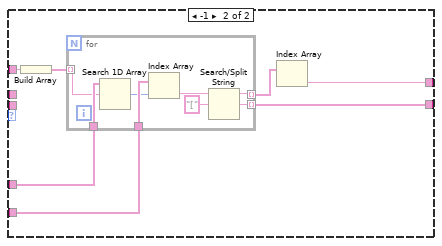
[diagram p13: hidden frame]
diagram:
  n1 = disable-structure shown="Enabled" {
    disable-tunnel: [w6 _] -> _
    disable-tunnel: [w7 _] -> _
    disable-tunnel: [w5 _] -> _
    frame Disabled {
      w12 = string[] ["Napetost generatorja faza R - G1 [kV]", "Napetost generatorja faza S - G1 [kV]", "Napetost generatorja faza T - G1 [kV]", "Tok generatorja faza R - G1 [kA]", "Tok generatorja faza S - G1 [kA]", "Tok generatorja faza T - G1 [kA]", "Napetost rotorja generatorja - G1 [V]", "Tok rotorja generatorja - G1 [A]", "Napetost za blok transformatorjem faza R - G1 [kV]", "Napetost za blok transformatorjem faza S - G1 [kV]", "Napetost za blok transformatorjem faza T - G1 [kV]", "Tok za blok transformatorjem faza R - G1 [A]", "Tok za blok transformatorjem faza S - G1 [A]", "Tok za blok transformatorjem faza T - G1 [A]", "Napetost generatorja faza R - G2 [kV]", "Napetost generatorja faza S - G2 [kV]", "Napetost generatorja faza T - G2 [kV]", "Tok generatorja faza R - G2 [kA]", "Tok generatorja faza S - G2 [kA]", "Tok generatorja faza T - G2 [kA]", "Napetost rotorja generatorja - G2 [V]", "Tok rotorja generatorja - G2 [A]", "Napetost za blok transformatorjem faza R - G2 [kV]", "Napetost za blok transformatorjem faza S - G2 [kV]", "Napetost za blok transformatorjem faza T - G2 [kV]", "Tok za blok transformatorjem faza R - G2 [A]", "Tok za blok transformatorjem faza S - G2 [A]", "Tok za blok transformatorjem faza T - G2 [A]", "Napetost generatorja faza R - G3 [kV]", "Napetost generatorja faza S - G3 [kV]", "Napetost generatorja faza T - G3 [kV]", "Tok generatorja faza R - G3 [kA]", "Tok generatorja faza S - G3 [kA]", "Tok generatorja faza T - G3 [kA]", "Napetost rotorja generatorja - G3 [V]", "Tok rotorja generatorja - G3 [A]", "Napetost za blok transformatorjem faza R - G3 [kV]", "Napetost za blok transformatorjem faza S - G3 [kV]", "Napetost za blok transformatorjem faza T - G3 [kV]", "Tok za blok transformatorjem faza R - G3 [A]", "Tok za blok transformatorjem faza S - G3 [A]", "Tok za blok transformatorjem faza T - G3 [A]"]  # Waveform Name
      w17 = "codis_cli" ("userID")
      # ">>NAMES>>"
      # ">>LABELS>>"
      n2 = call-poly <vilib>:"DB Tools Open Connection.vi"("password"=w17, "userID"=w17, "connection information"="codis-dm_unit2_doblar" ("userID")) -> ("error out"=w18:errorcluster, "connection reference"=w19:T1)  [unwired: 5 in]
      n3 = call "Read_tSignal_Core.vi"("error in (no error)"=w18, "connection reference IN"=w19) -> ("error out"=w14:errorcluster, "SignalLabel OUT"=w6:string[], "connection reference OUT"=w15:T1, "idtSignal OUT"=w5:u16[])  [unwired: 5 in, 1 out]
      n4 = call "Read_tSensor_Core.vi"("error in (no error)"=w14, "connection reference IN"=w15) -> ("SensorLabel OUT"=w11:string[], "SensorNameUnit OUT"=w13:string[])  [unwired: 5 in, 3 out]
      n5 = Build Array (concatenate)(w11, string[] ["VOL000", "VOL001", "VOL002", "CURR000", "CURR001", "CURR002", "VOL003", "CURR003", "VOL004", "VOL005", "VOL006", "CURR004", "CURR005", "CURR006"]) -> (w8:string[])
      n6 = Build Array (concatenate)(w13, w12) -> (w9:string[])
      n7 = for {
        tunnel: w6 -> [w22] mode=indexing
        tunnel: [w24] -> w7 mode=indexing
        tunnel: w8 -> [w21]
        tunnel: w9 -> [w20]
        n8 = Search/Split String(string=w22, search string/char (-)=".") -> (substring before match=w26:string, match + rest of string=w25:string, offset of match=w23:i32)  [unwired: 1 in]
        n9 = case shown="0, Default" w23 {
          tunnel: w26 -> [w28 _]
          tunnel: w25 -> [w31 _]
          tunnel: [w35 w109] -> w24
          tunnel: w22 -> [_ w109]
          tunnel: w21 -> [w34 _]
          tunnel: w20 -> [w33 _]
          frame 0, Default {
            n10 = Search/Split String(string=w28, search string/char (-)="&") -> (substring before match=w38:string, match + rest of string=w37:string, offset of match=w39:i32)  [unwired: 1 in]
            n11 = case shown="0, Default" w39 {
              tunnel: w28 -> [_ w100]
              tunnel: [w74 w99] -> w36
              tunnel: w38 -> [w78 _]
              tunnel: w37 -> [w73 _]
              tunnel: w34 -> [w66 w98]
              tunnel: w33 -> [w65 w97]
              tunnel: [w64 w94] -> w30
              tunnel: w31 -> [_ _]
              frame 0, Default {
                n12 = Build Array(w78) -> (w70:string[])
                n13 = String Subset(string=w73, offset (0)=1) -> (substring=w71:string)  [unwired: 1 in]
                n14 = Build Array(w71) -> (w68:string[])
                n15 = for {
                  tunnel: w70 -> [w92] mode=indexing
                  tunnel: w66 -> [w93]
                  tunnel: w65 -> [w91]
                  tunnel: [w87] -> w69 mode=indexing
                  tunnel: [w86] -> w64 mode=indexing
                  n16 = Search 1D Array(1D array=w93, element=w92) -> (index of element=w90:i32)  [unwired: 1 in]
                  n17 = Index Array(array=w91, index=w90) -> (element=w88:string)
                  n18 = Search/Split String(string=w88, search string/char (-)="[") -> (substring before match=w87:string, match + rest of string=w86:string)  [unwired: 1 in, 1 out]
                }
                n19 = for {
                  tunnel: w68 -> [w84] mode=indexing
                  tunnel: w66 -> [w85]
                  tunnel: w65 -> [w83]
                  tunnel: [w79] -> w67 mode=indexing
                  n20 = Search 1D Array(1D array=w85, element=w84) -> (index of element=w82:i32)  [unwired: 1 in]
                  n21 = Index Array(array=w83, index=w82) -> (element=w80:string)
                  n22 = Search/Split String(string=w80, search string/char (-)="[") -> (substring before match=w79:string)  [unwired: 1 in, 2 out]
                }
                n23 = Index Array(array=w69) -> (element=w77:string)  [unwired: 1 in]
                n24 = Index Array(array=w67) -> (element=w76:string)  [unwired: 1 in]
                n25 = Concatenate Strings(w77, "&" ("search string/char (-)"), w76) -> (w74:string)
              }
              frame -1 {
                n26 = Build Array(w100) -> (w96:string[])
                n27 = for {
                  tunnel: w96 -> [w107] mode=indexing
                  tunnel: w98 -> [w108]
                  tunnel: w97 -> [w106]
                  tunnel: [w102] -> w95 mode=indexing
                  tunnel: [w101] -> w94 mode=indexing
                  n28 = Search 1D Array(1D array=w108, element=w107) -> (index of element=w105:i32)  [unwired: 1 in]
                  n29 = Index Array(array=w106, index=w105) -> (element=w104:string)
                  n30 = Search/Split String(string=w104, search string/char (-)="[") -> (substring before match=w102:string, match + rest of string=w101:string)  [unwired: 1 in, 1 out]
                }
                n31 = Index Array(array=w95) -> (element=w99:string)  [unwired: 1 in]
              }
            }
            n32 = case shown="\".CosFi\"" w31 {
              selector: w31 -> [w43 _ _ _ _ _]
              tunnel: w30 -> [w47 _ _ _ _ w59]
              tunnel: [w41 string[] ["[Hz]"] string[] ["[%]"] string[] ["[%]"] string[] ["[°]"] w58] -> w29
              tunnel: w28 -> [_ _ _ _ _ w57]
              frame "", Default {
                n33 = Search/Split String(string=w43, search string/char (-)="Ph") -> (offset of match=w46:i32)  [unwired: 1 in, 2 out]
                n34 = case shown="0, Default" w46 {
                  tunnel: w47 -> [_ w52]
                  tunnel: [string[] ["[°]"] w52] -> w42
                  frame 0, Default {
                  }
                  frame -1 {
                  }
                }
                n35 = Search/Split String(string=w43, search string/char (-)="PoleNum") -> (offset of match=w45:i32)  [unwired: 1 in, 2 out]
                n36 = case shown="0, Default" w45 {
                  tunnel: w42 -> [_ w50]
                  tunnel: [string[] ["[Number]"] w50] -> w41
                  frame 0, Default {
                  }
                  frame -1 {
                  }
                }
              }
              frame ".SignalFrequency" {
              }
              frame ".CosFi" {
              }
              frame ".THD", ".TotalTHD" {
              }
              frame ".PhaseDifference" {
              }
              frame ".DC" {
                n37 = Search/Split String(string=w57, search string/char (-)="TRG") -> (offset of match=w60:i32)  [unwired: 1 in, 2 out]
                n38 = case shown="0, Default" w60 {
                  tunnel: w59 -> [_ w63]
                  tunnel: [string[] ["[V]"] w63] -> w58
                  frame 0, Default {
                  }
                  frame -1 {
                  }
                }
              }
            }
            n39 = Concatenate Strings(w36, w31, "." ("search string/char (-)"), w29) -> (w35:string)
          }
          frame -1 {
          }
        }
      }
    }
    frame Enabled {
    }
  }
  n40 = for {
    tunnel: "SignalNames" -> [w113] mode=indexing
    tunnel: [w110] -> w1 mode=indexing
    n41 = Search and Replace String(input string=w113, search string="G1", replace string="G1" ("search string")) -> (result string=w110:string)  [unwired: 5 in, 3 out]
  }
  n42 = disable-structure shown="Enabled" {
    disable-tunnel: "SignalLabels" -> [w126 _]
    disable-tunnel: w1 -> [w125 _]
    disable-tunnel: "idtSignal OUT" -> [w114 _]
    frame Enabled {
      w115 = "codis_cli" ("userID")
      n43 = for {
        tunnel: w126 -> [w139] mode=indexing
        tunnel: [w137] -> w121 mode=indexing
        tunnel: w125 -> [w134] mode=indexing
        tunnel: w114 -> [w133] mode=indexing
        i -> [w136]
        n44 = disable-structure shown="Enabled" {
          disable-tunnel: w136 -> [w142 _]
          disable-tunnel: [w140 w143] -> w135
          disable-tunnel: w133 -> [_ w143]
          frame Disabled {
            n45 = Add(x=0, y=w142) -> (x+y=w140:i32)
          }
          frame Enabled {
          }
        }
        n46 = Bundle("data"=w135, "data"=w139, "result string"=w134, "String"="") -> (w137:T2)  [unwired: 1 in]
      }
      n47 = call-poly <vilib>:"DB Tools Open Connection.vi"("password"=w115, "userID"=w115, "connection information"="codis-dm_unit1_doblar" ("userID")) -> ("error out"=w123:errorcluster, "connection reference"=w124:T1)  [unwired: 5 in]
      n48 = for {
        tunnel: w124 -> [w132]
        tunnel: w123 -> [w131]
        tunnel: "tsignal" ("table") -> [w130]
        tunnel: w121 -> [w129] mode=indexing
        tunnel: [w128] -> w117
        tunnel: [w127] -> w118
        tunnel: string[] ["idtSignal", "SignalLabel", "SignalNameUnit", "SignalDescription"] ("columns") -> [_]
        n49 = call <vilib>:"DB Tools Insert Data.vi"("data"=w129, "error in (no error)"=w131, "table"=w130, "connection reference"=w132) -> ("error out"=w128:errorcluster, "connection reference out"=w127:T1)  [unwired: 6 in]
      }
      n50 = call <vilib>:"DB Tools Close Connection.vi"("error in (no error)"=w117, "connection reference"=w118) -> ("error out"=→"error out":errorcluster)  [unwired: 5 in]
    }
    frame Disabled {
    }
  }
